vi "http parse function.vi"(9 "transmit queue":refnum<queue>, 10 "data in":string, 11 "application request in":T1) -> (2 "abort":bool, 3 "application request out":T1)   [LabVIEW 2013]
uses:
  http response.ctl
  http response packet type.ctl
  http request.ctl
  http method.ctl
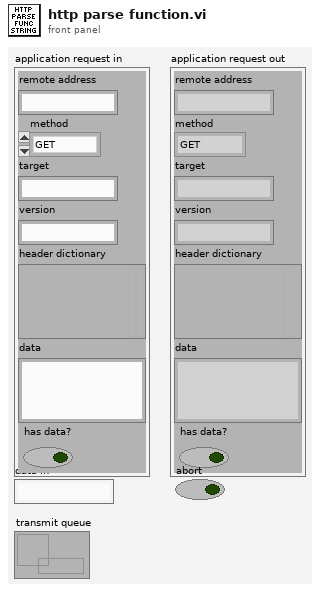
[diagram p1: front panel]
types:
  T1 = typedef "http request.ctl" = cluster{"remote address":string, "method":T2, "target":string, "version":string, "header dictionary":variant, "data":string, "has data?":bool}
  T2 = typedef "http method.ctl" = enum16{"GET", "POST", "PUT", "DELETE", "HEAD", "OPTIONS"}
  T3 = typedef "http response.ctl" = cluster{"packet type":T4, "version":string, "reason code":u16, "status string":string, "header dictionary":variant, "cookies":string[], "data":string}
  T4 = typedef "http response packet type.ctl" = enum16{"full response", "header only", "data only", "last data"}
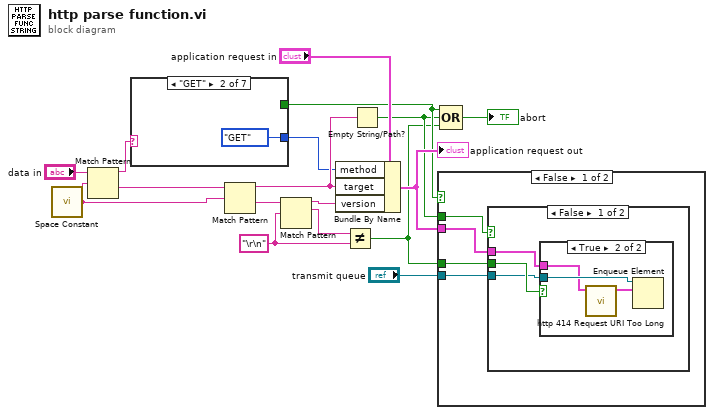
[diagram p0: block diagram]
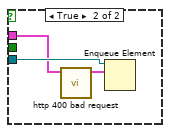
[diagram p3: hidden frame]
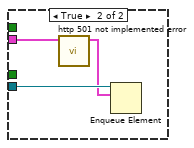
[diagram p4: hidden frame]
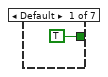
[diagram p5: hidden frame]
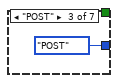
[diagram p6: hidden frame]
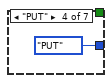
[diagram p7: hidden frame]
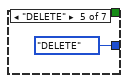
[diagram p8: hidden frame]
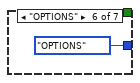
[diagram p9: hidden frame]
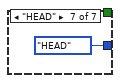
[diagram p10: hidden frame]
diagram:
  w5 = "\r\n"
  n1 = call <vilib>:"Space Constant.vi"() -> ("String"=w12:string)
  n2 = Match Pattern(string="data in", regular expression=w12) -> (before substring=w13:string, after substring=w10:string)  [unwired: 1 in, 2 out]
  n3 = case shown="\"GET\"" w13 {
    tunnel: [TRUE _ _ _ _ _ _] -> w6
    tunnel: [_ http_method."GET" ("method") http_method."POST" ("method") http_method."PUT" ("method") http_method."DELETE" ("method") http_method."OPTIONS" ("method") http_method."HEAD" ("method")] -> w15
    frame Default {
    }
    frame "GET" {
    }
    frame "POST" {
    }
    frame "PUT" {
    }
    frame "DELETE" {
    }
    frame "OPTIONS" {
    }
    frame "HEAD" {
    }
  }
  n4 = Match Pattern(string=w10, regular expression=w12) -> (before substring=w16:string, after substring=w11:string)  [unwired: 1 in, 2 out]
  n5 = Match Pattern(string=w11, regular expression=w5) -> (before substring=w17:string, match substring=w4:string)  [unwired: 1 in, 2 out]
  n6 = Bundle By Name(cluster="application request in", "method"=w15, "target"=w16, "version"=w17) -> (w7:T1)
  "application request out" <- w7
  n7 = Not Equal?(x=w4, y=w5) -> (x != y?=w1:bool)
  n8 = Empty String/Path?(string/path=w16) -> (empty?=w2:bool)
  n9 = case shown="False" w6 {
    tunnel: w7 -> [w26 w40]
    tunnel: "transmit queue" -> [w27 w39]
    tunnel: w2 -> [w28 _]
    tunnel: w1 -> [w25 _]
    frame False {
      n10 = case shown="False" w28 {
        tunnel: w27 -> [w30 w37]
        tunnel: w26 -> [w29 w35]
        tunnel: w25 -> [w31 _]
        frame False {
          n11 = case shown="True" w31 {
            tunnel: w30 -> [_ w34]
            tunnel: w29 -> [_ w32]
            frame False {
            }
            frame True {
              n12 = call "http 414 Request URI Too Long.vi"("application request in"=w32) -> ("application request out"=w33:T3)  [unwired: 10 in]
              n13 = Enqueue Element(queue=w34, element=w33) -> ()  [unwired: 2 in, 3 out]
            }
          }
        }
        frame True {
          n14 = call "http 400 bad request.vi"("application request in"=w35) -> ("application request out"=w36:T3)  [unwired: 10 in]
          n15 = Enqueue Element(queue=w37, element=w36) -> ()  [unwired: 2 in, 3 out]
        }
      }
    }
    frame True {
      n16 = call "http 501 not implemented error.vi"("application request in"=w40) -> ("application request out"=w38:T3)  [unwired: 10 in]
      n17 = Enqueue Element(queue=w39, element=w38) -> ()  [unwired: 2 in, 3 out]
    }
  }
  n18 = Compound Arithmetic op=OR(w6, w2, w1) -> (→"abort":bool)
